vi "UART_Initialize.vi"(0 "resource name":refnum<k15>="Digital1", 1 "timing file paths":path[](array[path]), 5 "pin map file":path caption="pin map file path", 7 "specifications file paths":path[](array[path]), 9 "patterns file paths":path[](array[path]), 11 "error in":errorcluster, 12 "levels file paths":path[](array[path])) -> (4 "instrument handle out":refnum<k15>, 15 "error out":errorcluster)   [LabVIEW 2024, in "UART.lvlib"]
doc: "Initialized NI PXIe-657x board.\nSet Pinmap, Timing files, Level files, Specification fils and Patterns.\nAll the channels are set to Digital function"
uses:
  UART.lvlib
  <instrlib>/niDigital/niDigital.llb/niDigital Selected Function.ctl
  <instrlib>/niDigital/niDigital.llb/niDigital Load Specifications Levels and Timing (Multiple).vi
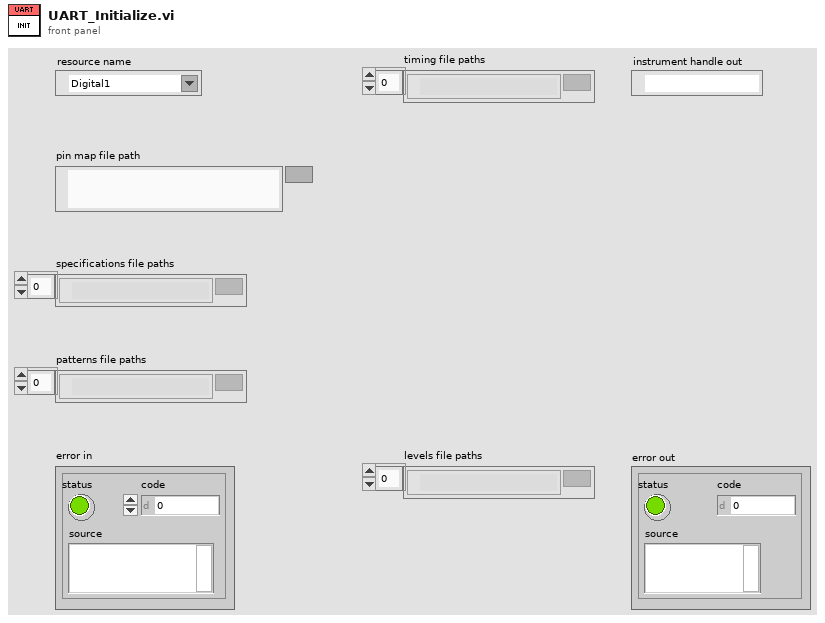
[diagram p1: front panel]
types:
  T1 = typedef "niDigital Selected Function.ctl" = i32
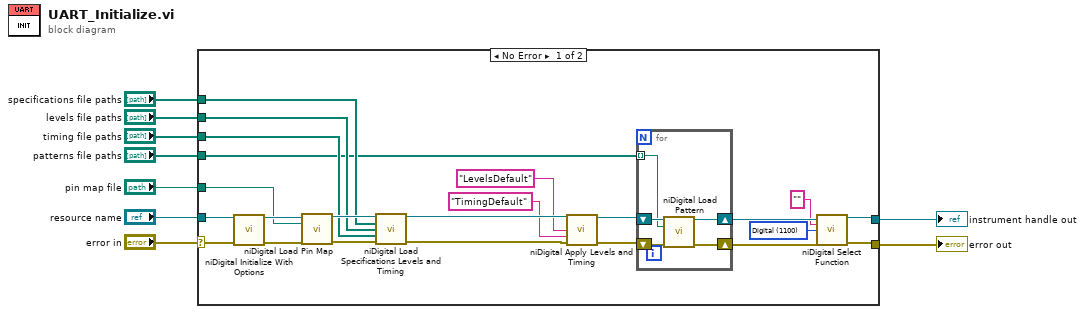
[diagram p0: block diagram]
diagram:
  n1 = case shown="No Error" "error in" {
    selector: "error in" -> [w23 w38]
    tunnel: "resource name" -> [w28 _]
    tunnel: "pin map file" -> [w27 _]
    tunnel: "specifications file paths" -> [w26 _]
    tunnel: "levels file paths" -> [w25 _]
    tunnel: "timing file paths" -> [w24 _]
    tunnel: [w13 w38] -> w4
    tunnel: [w12 _] -> w3
    tunnel: "patterns file paths" -> [w22 _]
    frame No Error {
      w11 = T1 1100 items=["Digital"=1100, "PPMU"=1101, "Off"=1102, "Disconnect"=1103, "RIO"=1104] ("function")
      n2 = call <instrlib>:"niDigital Initialize With Options.vi"("resource name"=w28, "error in"=w23) -> ("instrument handle"=w32:refnum<k15>, "error out"=w31:errorcluster)  [unwired: 12 in]
      n3 = call <instrlib>:"niDigital Load Pin Map.vi"("instrument handle"=w32, "pin map file"=w27, "error in"=w31) -> ("instrument handle out"=w30:refnum<k15>, "error out"=w29:errorcluster)  [unwired: 11 in]
      n4 = call-poly <instrlib>:"niDigital Load Specifications Levels and Timing.vi"("instrument handle"=w30, "specifications file paths"=w26, "levels file paths"=w25, "timing file paths"=w24, "error in"=w29) -> ("instrument handle out"=w18:refnum<k15>, "error out"=w21:errorcluster)  [unwired: 9 in]
      n5 = call <instrlib>:"niDigital Apply Levels and Timing.vi"("instrument handle"=w18, "levels sheet"="LevelsDefault", "timing sheet"="TimingDefault" ("levels sheet"), "error in"=w21) -> ("instrument handle out"=w19:refnum<k15>, "error out"=w20:errorcluster)  [unwired: 10 in]
      n6 = for {
        shift-right: [w34] -> w15
        shift-left: w20 -> [w37]
        shift-right: [w35] -> w14
        shift-left: w19 -> [w36]
        tunnel: w22 -> [w33] mode=indexing
        n7 = call <instrlib>:"niDigital Load Pattern.vi"("instrument handle"=w36, "pattern file"=w33, "error in"=w37) -> ("instrument handle out"=w35:refnum<k15>, "error out"=w34:errorcluster)  [unwired: 11 in]
      }
      n8 = call <instrlib>:"niDigital Select Function.vi"("instrument handle"=w14, "channel list"="", "function"=w11, "error in"=w15) -> ("instrument handle out"=w12:refnum<k15>, "error out"=w13:errorcluster)  [unwired: 10 in]
    }
    frame Error {
    }
  }
  "error out" <- w4
  "instrument handle out" <- w3
